vi "Сохр. рисунков мишеней в файл (SubVI).vi"(11 "error in":errorcluster, 13 "Кластер рисунков всех мишеней":T1) -> (14 "error out":errorcluster)   [LabVIEW 2013]
doc: "Сохранение рисунков мишеней в файл для последующего восстановления.."
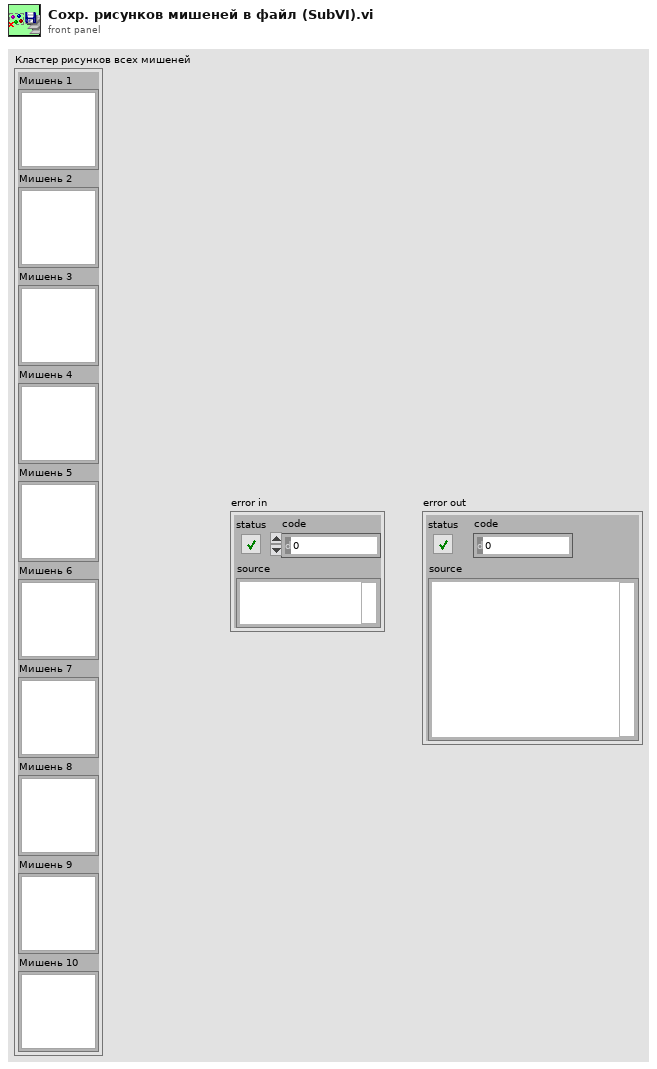
[diagram p1: front panel]
types:
  T1 = cluster{"Мишень 1":picture, "Мишень 2":picture, "Мишень 3":picture, "Мишень 4":picture, "Мишень 5":picture, "Мишень 6":picture, "Мишень 7":picture, "Мишень 8":picture, "Мишень 9":picture, "Мишень 10":picture}
  T2 = typedef "imagedata.ctl" = cluster{"image type":i32, "image depth":i32, "image":u8[], "mask":u8[], "colors":u32[], "Rectangle":cluster{"left":i16, "top":i16, "right":i16, "bottom":i16}}
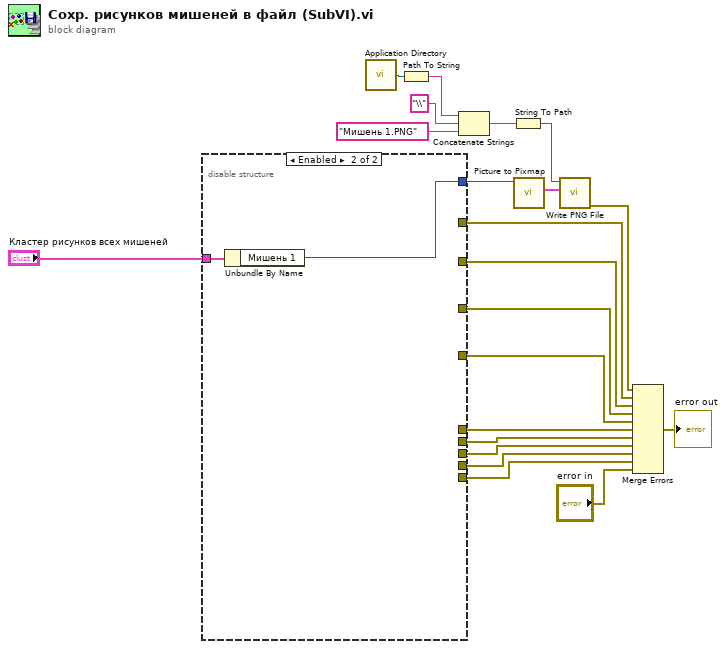
[diagram p0: block diagram]
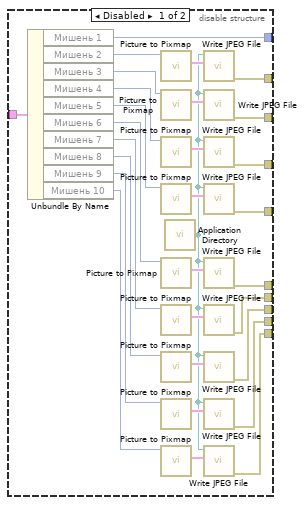
[diagram p2: hidden frame]
diagram:
  n1 = disable-structure shown="Enabled" {
    disable-tunnel: [w42 _] -> w20
    disable-tunnel: [w41 _] -> w19
    disable-tunnel: [w40 _] -> w18
    disable-tunnel: [w39 _] -> w17
    disable-tunnel: [w38 _] -> w16
    disable-tunnel: [w37 _] -> w15
    disable-tunnel: [w36 _] -> w14
    disable-tunnel: [w35 _] -> w13
    disable-tunnel: [w34 _] -> w12
    disable-tunnel: "Кластер рисунков всех мишеней" -> [w32 w53]
    disable-tunnel: [w31 w52] -> w10
    frame Disabled {
      n2 = Unbundle By Name(w32) -> ("Мишень 1"=w31:picture, "Мишень 2"=w30:picture, "Мишень 3"=w29:picture, "Мишень 4"=w28:picture, "Мишень 5"=w27:picture, "Мишень 6"=w26:picture, "Мишень 7"=w25:picture, "Мишень 8"=w24:picture, "Мишень 9"=w23:picture, "Мишень 10"=w22:picture)
      n3 = call <vilib>:"Picture to Pixmap.vi"("picture"=w30) -> ("image data"=w43:T2)  [unwired: 9 in, 1 out]
      n4 = call <vilib>:"Picture to Pixmap.vi"("picture"=w29) -> ("image data"=w44:T2)  [unwired: 9 in, 1 out]
      n5 = call <vilib>:"Picture to Pixmap.vi"("picture"=w28) -> ("image data"=w45:T2)  [unwired: 9 in, 1 out]
      n6 = call <vilib>:"Picture to Pixmap.vi"("picture"=w27) -> ("image data"=w46:T2)  [unwired: 9 in, 1 out]
      n7 = call <vilib>:"Picture to Pixmap.vi"("picture"=w26) -> ("image data"=w51:T2)  [unwired: 9 in, 1 out]
      n8 = call <vilib>:"Picture to Pixmap.vi"("picture"=w25) -> ("image data"=w50:T2)  [unwired: 9 in, 1 out]
      n9 = call <vilib>:"Picture to Pixmap.vi"("picture"=w24) -> ("image data"=w49:T2)  [unwired: 9 in, 1 out]
      n10 = call <vilib>:"Picture to Pixmap.vi"("picture"=w23) -> ("image data"=w48:T2)  [unwired: 9 in, 1 out]
      n11 = call <vilib>:"Picture to Pixmap.vi"("picture"=w22) -> ("image data"=w47:T2)  [unwired: 9 in, 1 out]
      n12 = call <vilib>:"Application Directory.vi"() -> ("Application Directory"=w33:path)
      n13 = call <vilib>:"Write JPEG File.vi"("image data"=w43, "path to JPEG file"=w33) -> ("error out"=w42:errorcluster)  [unwired: 8 in, 1 out]
      n14 = call <vilib>:"Write JPEG File.vi"("image data"=w44, "path to JPEG file"=w33) -> ("error out"=w41:errorcluster)  [unwired: 8 in, 1 out]
      n15 = call <vilib>:"Write JPEG File.vi"("image data"=w45, "path to JPEG file"=w33) -> ("error out"=w40:errorcluster)  [unwired: 8 in, 1 out]
      n16 = call <vilib>:"Write JPEG File.vi"("image data"=w46, "path to JPEG file"=w33) -> ("error out"=w39:errorcluster)  [unwired: 8 in, 1 out]
      n17 = call <vilib>:"Write JPEG File.vi"("image data"=w51, "path to JPEG file"=w33) -> ("error out"=w38:errorcluster)  [unwired: 8 in, 1 out]
      n18 = call <vilib>:"Write JPEG File.vi"("image data"=w50, "path to JPEG file"=w33) -> ("error out"=w37:errorcluster)  [unwired: 8 in, 1 out]
      n19 = call <vilib>:"Write JPEG File.vi"("image data"=w49, "path to JPEG file"=w33) -> ("error out"=w36:errorcluster)  [unwired: 8 in, 1 out]
      n20 = call <vilib>:"Write JPEG File.vi"("image data"=w48, "path to JPEG file"=w33) -> ("error out"=w35:errorcluster)  [unwired: 8 in, 1 out]
      n21 = call <vilib>:"Write JPEG File.vi"("image data"=w47, "path to JPEG file"=w33) -> ("error out"=w34:errorcluster)  [unwired: 8 in, 1 out]
    }
    frame Enabled {
      n22 = Unbundle By Name(w53) -> ("Мишень 1"=w52:picture)
    }
  }
  n23 = call <vilib>:"Application Directory.vi"() -> ("Application Directory"=w3:path)
  n24 = Path To String(path=w3) -> (string=w4:string)
  n25 = Concatenate Strings(w4, "\\" ("string"), "Мишень 1.PNG" ("string")) -> (w7:string)
  n26 = String To Path(string=w7) -> (path=w2:path)
  n27 = call <vilib>:"Picture to Pixmap.vi"("picture"=w10) -> ("image data"=w21:T2)  [unwired: 9 in, 1 out]
  n28 = call <vilib>:"Write PNG File.vi"("image data"=w21, "path to PNG file"=w2) -> ("error out"=w1:errorcluster)  [unwired: 8 in, 1 out]
  n29 = Merge Errors(w1, w20, w19, w18, w17, w16, w15, w14, w13, w12, "error in") -> (→"error out":errorcluster)
